vi "READ SONAR.vi"(6 "Range Units":T4, 7 "ping time (s)":sgl=1e-05, 8 "error in (no error)":errorcluster, 10 "SONAR refname":string, 11 "SonarSRF04DevRef":T1) -> (0 "error out":errorcluster, 3 "Distance":dbl)   [LabVIEW 2020]
uses:
  <vilib>/Rock Robotics/WPI/Ultrasonic/WPI_SonarSRF04DigitalGetRange.vi
  <vilib>/Rock Robotics/Network Tables/NT Write Number.vi
  <vilib>/Rock Robotics/SystemInterfaces/DIO/FPGA_DIOChannel.ctl
  <vilib>/Rock Robotics/SystemInterfaces/Counter/FPGA_CounterCtrSystemIndex.ctl
  <vilib>/Rock Robotics/WPI/Ultrasonic/WPI_UltrasonicDeviceRef.ctl
  <vilib>/Rock Robotics/WPI/Ultrasonic/WPI_UltrasonicRangeUnits.ctl
panel:
  out "UltrasonicDevRef":T1={"DevStatus"={"status"=FALSE, "code"=0, "source"=""}, "Ping Channel"=enum."Invalid", "Echo Channel"=enum."Invalid", "CntIndex"=enum."Invalid"}
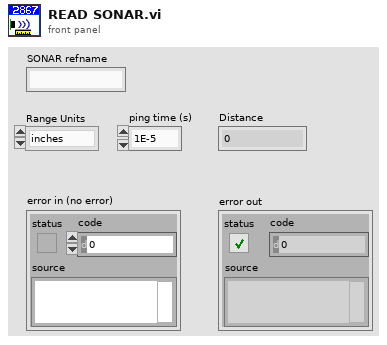
[diagram p1: front panel]
types:
  T1 = typedef "WPI_UltrasonicDeviceRef.ctl" = cluster{"DevStatus":errorcluster, "Ping Channel":T2, "Echo Channel":T2, "CntIndex":T3}
  T2 = typedef "FPGA_DIOChannel.ctl" = enum8{"DIO 0", "DIO 1", "DIO 2", "DIO 3", "DIO 4", "DIO 5", "DIO 6", "DIO 7", "DIO 8", "DIO 9", "DIO MXP 0", "DIO MXP 1", "DIO MXP 2", "DIO MXP 3", "DIO MXP 4", "DIO MXP 5", "DIO MXP 6", "DIO MXP 7", "DIO MXP 8", "DIO MXP 9", "DIO MXP 10", "DIO MXP 11", "DIO MXP 12", "DIO MXP 13", "DIO MXP 14", "DIO MXP 15", "SPI Port CS1", "SPI Port CS2", "SPI Port CS3", "SPI Port MISO", "SPI Port MOSI", "Invalid"}
  T3 = typedef "FPGA_CounterCtrSystemIndex.ctl" = enum8{"Ctr 0", "Ctr 1", "Ctr 2", "Ctr 3", "Ctr 4", "Ctr 5", "Ctr 6", "Ctr 7", "Invalid"}
  T4 = typedef "WPI_UltrasonicRangeUnits.ctl" = enum16{"inches", "mm"}
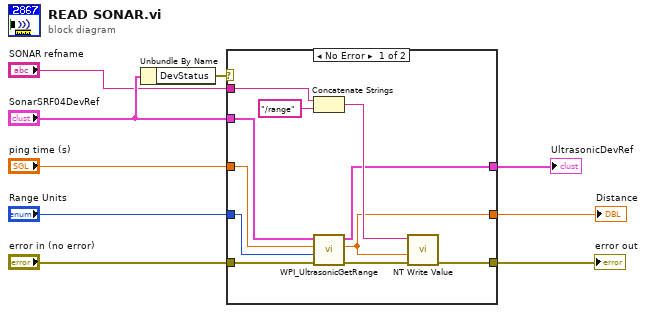
[diagram p0: block diagram]
diagram:
  n1 = Unbundle By Name("SonarSRF04DevRef") -> ("DevStatus"=w8:errorcluster)
  n2 = case shown="No Error" w8 {
    tunnel: "SONAR refname" -> [w17 _]
    tunnel: "SonarSRF04DevRef" -> [w16 _]
    tunnel: "error in (no error)" -> [w15 _]
    tunnel: "Range Units" -> [w14 _]
    tunnel: [w13 _] -> w4
    tunnel: [w12 _] -> w3
    tunnel: "ping time (s)" -> [w11 _]
    tunnel: [w10 _] -> w1
    frame No Error {
      n3 = Concatenate Strings(w17, "/range" ("string")) -> (w20:string)
      n4 = call-poly <vilib>:"WPI_UltrasonicGetRange.vi"("error in (no error)"=w15, "Range Units"=w14, "ping time (s)"=w11, "UltrasonicDevRef"=w16) -> ("error out"=w18:errorcluster, "Distance"=w12:dbl, "UltrasonicDevRef"=w10:T1)  [unwired: 5 in]
      n5 = call-poly <vilib>:"NT Write Value.vi"("error in"=w18, "Numeric"=w12, "Name"=w20) -> ("error out"=w13:errorcluster)  [unwired: 8 in]
    }
    frame Error {
    }
  }
  "error out" <- w4
  "Distance" <- w3
  "UltrasonicDevRef" <- w1
